vi "add_ref_obj.vi"(1 "input cluster":T1) -> (0 "output cluster":T2)   [LabVIEW 2010]
uses:
  MWT_1.3.0_r1035/MultiWorm Tracker v1.3.0/data/MWT.dll
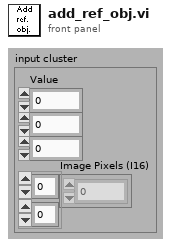
[diagram p1: front panel]
types:
  T1 = cluster{"Value":i32, i32, i32, "Image Pixels (I16)":i16[][]}
  T2 = cluster{"return type":i32, "return type":i32, "image":i16[][]}
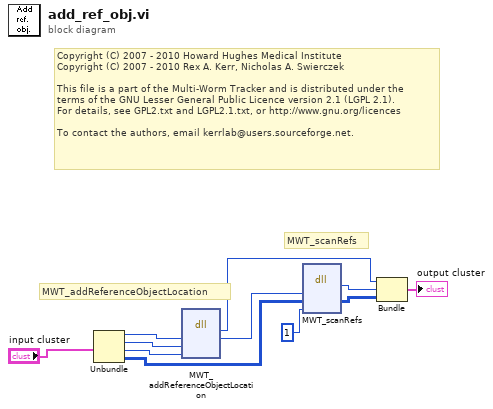
[diagram p0: block diagram]
diagram:
  # "Copyright (C) 2007 - 2010 Howard Hughes Medical Institute\nCopyright (C) 2007 - 2010 Rex A. Kerr, Nicholas A. Swierczek\n \nThis file is a part of the Multi-Worm Tracker and is distributed under the\nterms of the GNU Lesser General Public Licence version 2.1 (LGPL 2.1).\nFor details, see GPL2.txt and LGPL2.1.txt, or http://www.gnu.org/licences\n \nTo contact the authors, email kerrlab@users.sourceforge.net."
  # "MWT_scanRefs"
  # "MWT_addReferenceObjectLocation"
  n1 = Unbundle("input cluster") -> ("Value"=w10:i32, w8:i32, w7:i32, "Image Pixels (I16)"=w9:i16[][])
  n2 = dll-call lib="C:/Users/Marc/multi worm tracker/MWT_1.3.0_r1035/MultiWorm Tracker v1.3.0/data/MWT.dll" fn="MWT_addReferenceObjectLocation"("handle"=w10, "x"=w8, "y"=w7) -> ("return type"=w4:i32, "handle"=w11:i32)  [unwired: 5 in, 2 out]
  n3 = dll-call lib="C:/Users/Marc/multi worm tracker/MWT_1.3.0_r1035/MultiWorm Tracker v1.3.0/data/MWT.dll" fn="MWT_scanRefs"("handle"=w11, "image"=w9, "bin"=1) -> ("return type"=w5:i32, "image"=w6:i16[][])  [unwired: 5 in, 2 out]
  n4 = Bundle("return type"=w4, "return type"=w5, "image"=w6) -> (→"output cluster":T2)  [unwired: 1 in]
